vi "ICM Calculate Records.vi"(9 "Assemble?":bool, 11 "Stream Data":string) -> (1 "Data":T1(array[cluster]), 3 "# of Records":i32)   [LabVIEW 2018]
doc: "OSDS Calculate Records.vi\n\n This VI calculates the number of records contained in the binary string of data from a Stream file.\n\nOCC Streaming Data System Version 1.0\nJune, 2007 Original Code Consulting David Thomson\n www.originalcode.com"
panel:
  out "Array 3":string[](array[string])
  out "Array 2":string[](array[string])
  out "Array":i32[](array[numeric])
  out "Records OK?":bool
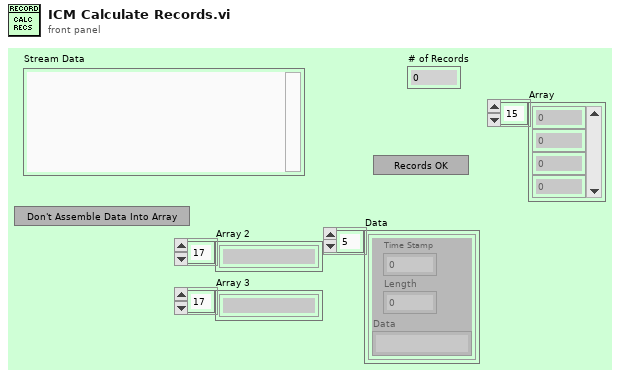
[diagram p1: front panel]
types:
  T1 = cluster{"Time Stamp":dbl, "Length":i32, "Data":string}[]
  T2 = cluster{"Time Stamp":dbl, "Length":i32, "Stream Data":string}[]
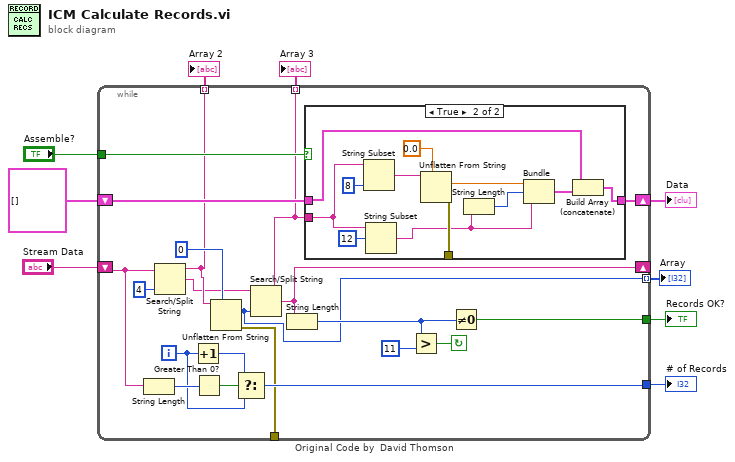
[diagram p0: block diagram]
diagram:
  n1 = while "Original Code by  David Thomson" {
    shift-right: [w17] -> _
    shift-left: "Stream Data" -> [w10]
    tunnel: [w22] -> w8
    tunnel: [w21] -> w7
    tunnel: "Assemble?" -> [w20]
    shift-right: [w19] -> w4
    shift-left: T1 [] -> [w18]
    tunnel: [w16] -> _
    tunnel: [w14] -> w3 mode=indexing
    tunnel: [w13] -> w2 mode=indexing
    tunnel: [w11] -> w1 mode=indexing
    i -> [w23]
    stop <- w28 continue-if-true
    n2 = String Length(string=w10) -> (length=w26:i32)
    n3 = Search/Split String(string=w10, offset (0)=4) -> (substring before match=w13:string, match + rest of string=w12:string)  [unwired: 2 out]
    n4 = Increment(x=w23) -> (x+1=w24:i32)
    n5 = Greater Than 0?(x=w26) -> (x > 0?=w25:bool)
    n6 = Unflatten From String(type=0 ("offset (0)"), binary string=w13) -> (value=w14:i32, error out=w16:errorcluster)  [unwired: 1 in, 3 out]
    n7 = Select(t=w24, s=w25, f=w23) -> (s? t:f=w22:i32)
    n8 = Search/Split String(string=w12, offset (0)=w14) -> (substring before match=w11:string, match + rest of string=w17:string)  [unwired: 2 out]
    n9 = String Length(string=w17) -> (length=w27:i32)
    n10 = case shown="True" w20 {
      tunnel: [w31 w38] -> w19
      tunnel: w18 -> [w31 w37]
      tunnel: w11 -> [_ w33]
      tunnel: [_ w35] -> _
      frame False {
      }
      frame True {
        n11 = String Subset(string=w33, length (rest)=8 ("length (rest)")) -> (substring=w42:string)  [unwired: 1 out]
        n12 = String Subset(string=w33, offset (0)=12) -> (substring=w32:string)  [unwired: 1 out]
        n13 = Unflatten From String(type=0.0, binary string=w42) -> (value=w41:dbl, error out=w35:errorcluster)  [unwired: 1 in, 3 out]
        n14 = String Length(string=w32) -> (length=w40:i32)
        n15 = Bundle(w41, w40, "Stream Data"=w32) -> (w39:cluster{dbl, i32, "Stream Data":string})  [unwired: 1 out]
        n16 = Build Array (concatenate)(w37, w39) -> (w38:T2)
      }
    }
    n17 = Greater?(x=w27, y=11) -> (0:w28:bool)
    n18 = Not Equal To 0?(x=w27) -> (x != 0?=w21:bool)
  }
  "# of Records" <- w8
  "Records OK?" <- w7
  "Data" <- w4
  "Array" <- w3
  "Array 2" <- w2
  "Array 3" <- w1
